vi "DefaultFromIni.vi"(8 "error in (no error)":errorcluster, 11 "RoomAlert in":refnum<class "RoomAlert.lvclass">) -> (0 "error out":errorcluster, 3 "RoomAlert out":refnum<class "RoomAlert.lvclass">)   [LabVIEW 2018, in "SensorPlugins.lvlib" / "RoomAlert.lvclass"]
doc: "Opens the configuration INI file and loads the information from the file into the class cluster."
uses:
  RoomAlert.lvclass
  C:/Program Files (x86)/National Instruments/LabVIEW 2018/user.lib/NIST/BaseClasses/BasePlugin_class/BasePlugin.lvclass
  TypeDefinitions/RoomAlertControls.ctl
  TypeDefinitions/MeasurementControls.ctl
  TypeDefinitions/MeasurementToRead.ctl
  <userlib>/NIST/BaseClasses/BasePlugin_class/BasePlugin.lvclass/BasePlugin.ctl
  <userlib>/NIST/BaseClasses/BasePlugin_class/Accessors/Read PluginIniFilePath.vi
  <vilib>/Utility/error.llb/Error Cluster From Error Code.vi
  <vilib>/ErrorRing/Error Ring.xnode
  <vilib>/Utility/config.llb/NI_LVConfig.lvlib
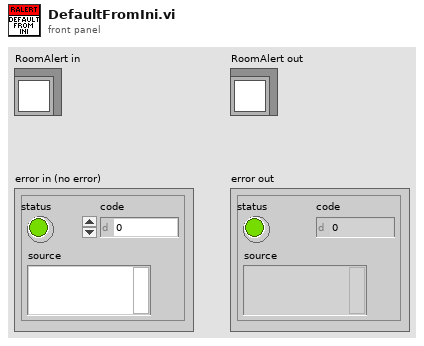
[diagram p1: front panel]
types:
  T1 = typedef "SensorPlugins.lvlib/RoomAlert.lvclass/MeasurementToRead.ctl" = cluster{"Type":string, "OID":string}[]
  T2 = typedef "SensorPlugins.lvlib/RoomAlert.lvclass/MeasurementControls.ctl" = cluster{"Measurement RefreshTime (ms)":u32, "Measurement Name":string, "Timeout(ms)":i32, "Amber Warning Light Configuration":cluster{"Warning Temperture (Degrees C)":dbl, "Temperature Delta (Degrees C/Minute)":dbl, "Time Window (Minutes)":dbl}}
  T3 = typedef "SensorPlugins.lvlib/RoomAlert.lvclass/RoomAlertControls.ctl" = cluster{"Connected?":bool, "IP Address of SNMP Device":string, "Port (161)":u16, "Community Name":string, "Measurements To Read Array":u16[], "Update LightTower?":bool, "LightTower":cluster{"Red":bool, "Amber":bool, "Green":bool, "Audio":bool}, "RoomAlert Model ID":string, "Sensor OID Numbers":string[][], "Sensor Light Tower OID Numbers":string[][]}[]
  T4 = typedef "NI_LVConfig.lvlib/Config Data RefNum.ctl" = refnum<k1>
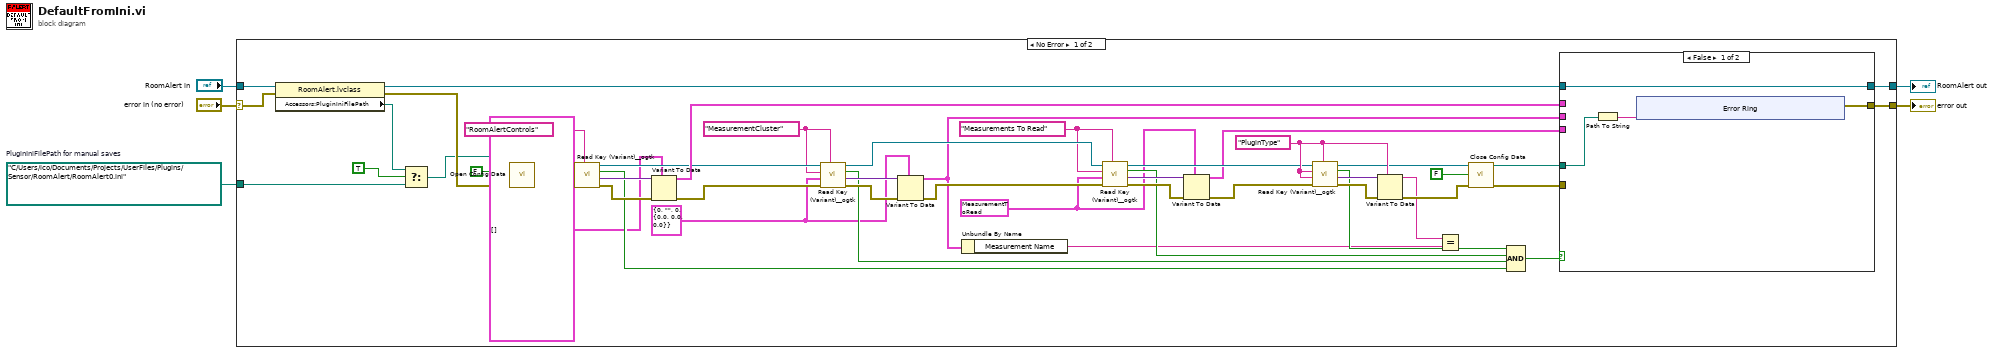
[diagram p0: block diagram]
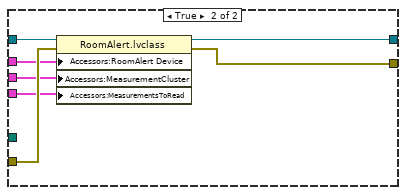
[diagram p2: hidden frame]
diagram:
  w1 = path "C:/Users/ico/Documents/Projects/UserFiles/Plugins/Sensor/RoomAlert/RoomAlert0.ini"  # PluginIniFilePath for manual saves
  n1 = case shown="No Error" "error in (no error)" {
    selector: "error in (no error)" -> [w53 w73]
    tunnel: "RoomAlert in" -> [w54 w74]
    tunnel: [w48 w74] -> w3
    tunnel: [w44 w73] -> w2
    tunnel: w1 -> [w14 _]
    frame No Error {
      w15 = T1 [{"Type"="Internal Temp F", "OID"="1.3.6.1.4.1.20916.1.6.1.1.1.1.0"}, {"Type"="Internal Temp C", "OID"="1.3.6.1.4.1.20916.1.6.1.1.1.2.0"}, {"Type"="Digital Sensor 1 Temp C", "OID"="1.3.6.1.4.1.20916.1.6.1.2.1.1.0"}, {"Type"="Digital Sensor 1 Temp F", "OID"="1.3.6.1.4.1.20916.1.6.1.2.1.2.0"}, {"Type"="Digital Sensor 2 Temp C", "OID"="1.3.6.1.4.1.20916.1.6.1.2.2.1.0"}, {"Type"="Digital Sensor 2 Temp F", "OID"="1.3.6.1.4.1.20916.1.6.1.2.2.2.0"}, {"Type"="Switch Sensor State", "OID"="1.3.6.1.4.1.20916.1.6.1.3.1.0"}, {"Type"="Signal Tower Red State", "OID"="1.3.6.1.4.1.20916.1.6.2.1.0"}, {"Type"="Signal Tower Amber State", "OID"="1.3.6.1.4.1.20916.1.6.2.2.0"}, {"Type"="Signal Tower Green State", "OID"="1.3.6.1.4.1.20916.1.6.2.3.0"}, {"Type"="Signal Tower Alarm 1", "OID"="1.3.6.1.4.1.20916.1.6.2.6.0"}, {"Type"="Alarm Message", "OID"="1.3.6.1.4.1.20916.1.6.3.1.0"}] ("MeasurementsToRead")
      w21 = "PluginType" ("section")
      w24 = T2 {"Measurement RefreshTime (ms)"=0, "Measurement Name"="", "Timeout(ms)"=0, "Amber Warning Light Configuration"={"Warning Temperture (Degrees C)"=0.0, "Temperature Delta (Degrees C/Minute)"=0.0, "Time Window (Minutes)"=0.0}} ("MeasurementCluster")
      w25 = T3 [] ("RoomAlert Device")
      w26 = "Measurements To Read" ("section")
      w32 = "MeasurementCluster" ("section")
      w41 = "RoomAlertControls" ("section")
      n2 = property class="RoomAlert.lvclass"(reference=w54, error in=w53) -> (reference out=w6:refnum<class "RoomAlert.lvclass">, error out=w51:errorcluster, "Accessors:PluginIniFilePath"=w12:path)
      n3 = Select(t=w12, s=TRUE ("Read from Property Node"), f=w14) -> (s? t:f=w11:path)
      n4 = call <vilib>:"Open Config Data.vi"("error in (no error)"=w51, "create file if necessary (T)"=FALSE, "configuration file path"=w11) -> ("error out"=w49:errorcluster, "refnum"=w50:T4)  [unwired: 6 in, 1 out]
      n5 = call <userlib>:"Read Key (Variant)__ogtk.vi"("section"=w41, "error in (no error)"=w49, "type"=w25, "key (optional)"=w41, "refnum"=w50) -> ("error out"=w46:errorcluster, "key-value"=w47:variant, "found?"=w39:bool, "refnum out"=w34:T4)  [unwired: 3 in]
      n6 = Variant To Data(error in=w46, type=w25, Variant=w47) -> (data=w45:T3, error out=w35:errorcluster)
      n7 = call <userlib>:"Read Key (Variant)__ogtk.vi"("section"=w32, "error in (no error)"=w35, "type"=w24, "key (optional)"=w32, "refnum"=w34) -> ("error out"=w37:errorcluster, "key-value"=w36:variant, "found?"=w33:bool, "refnum out"=w30:T4)  [unwired: 3 in]
      n8 = Variant To Data(error in=w37, type=w24, Variant=w36) -> (data=w9:T2, error out=w31:errorcluster)
      n9 = Unbundle By Name(w9) -> ("Measurement Name"=w7:string)
      n10 = call <userlib>:"Read Key (Variant)__ogtk.vi"("section"=w26, "error in (no error)"=w31, "type"=w15, "key (optional)"=w26, "refnum"=w30) -> ("error out"=w29:errorcluster, "key-value"=w28:variant, "found?"=w27:bool, "refnum out"=w18:T4)  [unwired: 3 in]
      n11 = Variant To Data(error in=w29, type=w15, Variant=w28) -> (data=w10:T1, error out=w19:errorcluster)
      n12 = call <userlib>:"Read Key (Variant)__ogtk.vi"("section"=w21, "error in (no error)"=w19, "type"=w21, "key (optional)"=w21, "refnum"=w18) -> ("error out"=w23:errorcluster, "key-value"=w22:variant, "found?"=w16:bool, "refnum out"=w17:T4)  [unwired: 3 in]
      n13 = Variant To Data(error in=w23, type=w21, Variant=w22) -> (data=w8:string, error out=w20:errorcluster)
      n14 = Equal?(x=w8, y=w7) -> ()  [unwired: 1 out]
      n15 = call <vilib>:"Close Config Data.vi"("error in (no error)"=w20, "write file if changed (T)"=FALSE, "refnum"=w17) -> ("error out"=w43:errorcluster, "file path"=w38:path)  [unwired: 7 in]
      n16 = Compound Arithmetic op=AND(w16, w27, w33, w39) -> (w40:bool)
      n17 = case shown="False" w40 {
        tunnel: w6 -> [w58 w72]
        tunnel: [w58 w69] -> w48
        tunnel: w45 -> [_ w70]
        tunnel: [w55 w68] -> w44
        tunnel: w43 -> [_ w71]
        tunnel: w38 -> [w56 _]
        tunnel: w9 -> [_ w67]
        tunnel: w10 -> [_ w66]
        frame False {
          n18 = Path To String(path=w56) -> (string=w57:string)
          n19 = xnode "Error Ring"("parameter 0"=w57) -> ("error out"=w55:errorcluster)
        }
        frame True {
          n20 = property class="RoomAlert.lvclass"(reference=w72, error in=w71, "Accessors:RoomAlert Device"=w70, "Accessors:MeasurementCluster"=w67, "Accessors:MeasurementsToRead"=w66) -> (reference out=w69:refnum<class "RoomAlert.lvclass">, error out=w68:errorcluster)
        }
      }
    }
    frame Error {
    }
  }
  "error out" <- w2
  "RoomAlert out" <- w3
